vi "004 shift register numero.vi"() -> ()   [LabVIEW 2019]
panel:
  out "Valor actual":dbl
  in  "increment":i32
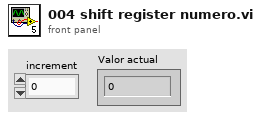
[diagram p1: front panel]
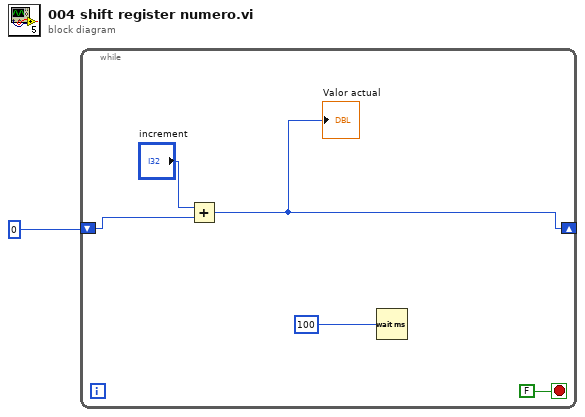
[diagram p0: block diagram]
diagram:
  n1 = while {
    shift-right: [w2] -> _
    shift-left: 0 -> [w4]
    stop <- FALSE stop-if-true
    n2 = Add(x="increment", y=w4) -> (x+y=w2:i32)
    "Valor actual" <- w2
    n3 = Wait (ms)(milliseconds to wait=u32 100 ("100")) -> ()  [unwired: 1 out]
  }
